vi "TDC_getDevType.vi"() -> (3 "Device Type":u16(ring) items=["quTAG", "None"])   [LabVIEW 2011]
uses:
  tdcbase.dll
panel:
  out "Error Out":errorcluster
  in  "Error In":errorcluster
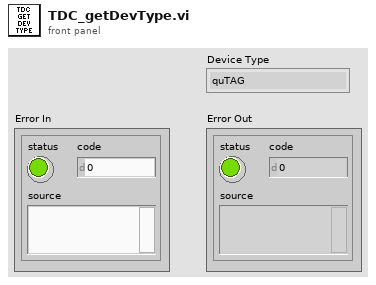
[diagram p1: front panel]
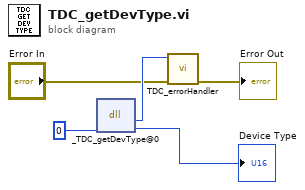
[diagram p0: block diagram]
diagram:
  n1 = dll-call lib="X:/tdcbase.dll" fn="_TDC_getDevType@0"("devType"=0) -> ("return type"=w3:i32, "devType"=→"Device Type":i32)  [unwired: 3 in, 2 out]
  n2 = call "TDC_errorHandler.vi"("Error In"="Error In", "TDC Return Code"=w3) -> ("Error Out"=→"Error Out":errorcluster)  [unwired: 9 in]
